vi "UnscentedKalmanFilter_Correct_OnlyUYR.vi"(4 "H_ExtraData":variant, 6 "H":T1, 7 "Rows":i32, 8 "R":T2, 9 "Y":T2, 10 "U":T2, 11 "in UnscentedKalmanFiilter":T3) -> (0 "Error":bool, 3 "out UnscentedKalmanFiilter":T3)   [LabVIEW 2019, in "Trajectory_Library.lvlib"]
doc: "Creates a new LINEAR SYSTEM data cluster with the specified values. \n\n\nInputs: \n - XXX -- XXX.\n\nOutputs:\n - XXX -- XXX."
uses:
  Trajectory_Library.lvlib
  UNSCENTED_KALMAN_FILTER.ctl
  <vilib>/Analysis/Matrix/Datatypes/RealMatrix.ctl
  MERWE_SCALED_SIGMA_PTS.ctl
  BiFunction_FUNC_TYPE.ctl
  <vilib>/Analysis/Matrix/NI_Matrix.lvlib
panel:
  # "<Inputs, 1>"
  # "<Rows, 1>"
  # "<Rows, Rows>"
  # "State Estimate <Statess,1>"
  # "<States, States>"
  # "<States, ?>"
  # "<Statess,  States>"
  # "<Outputs, Outputs>"
  # "<?, 1>"
  # "<?, 1>"
  # "State Estimate <Statess,1>"
  # "<States, States>"
  # "<States, ?>"
  # "<Statess,  States>"
  # "<Outputs, Outputs>"
  # "<?, 1>"
  # "<?, 1>"
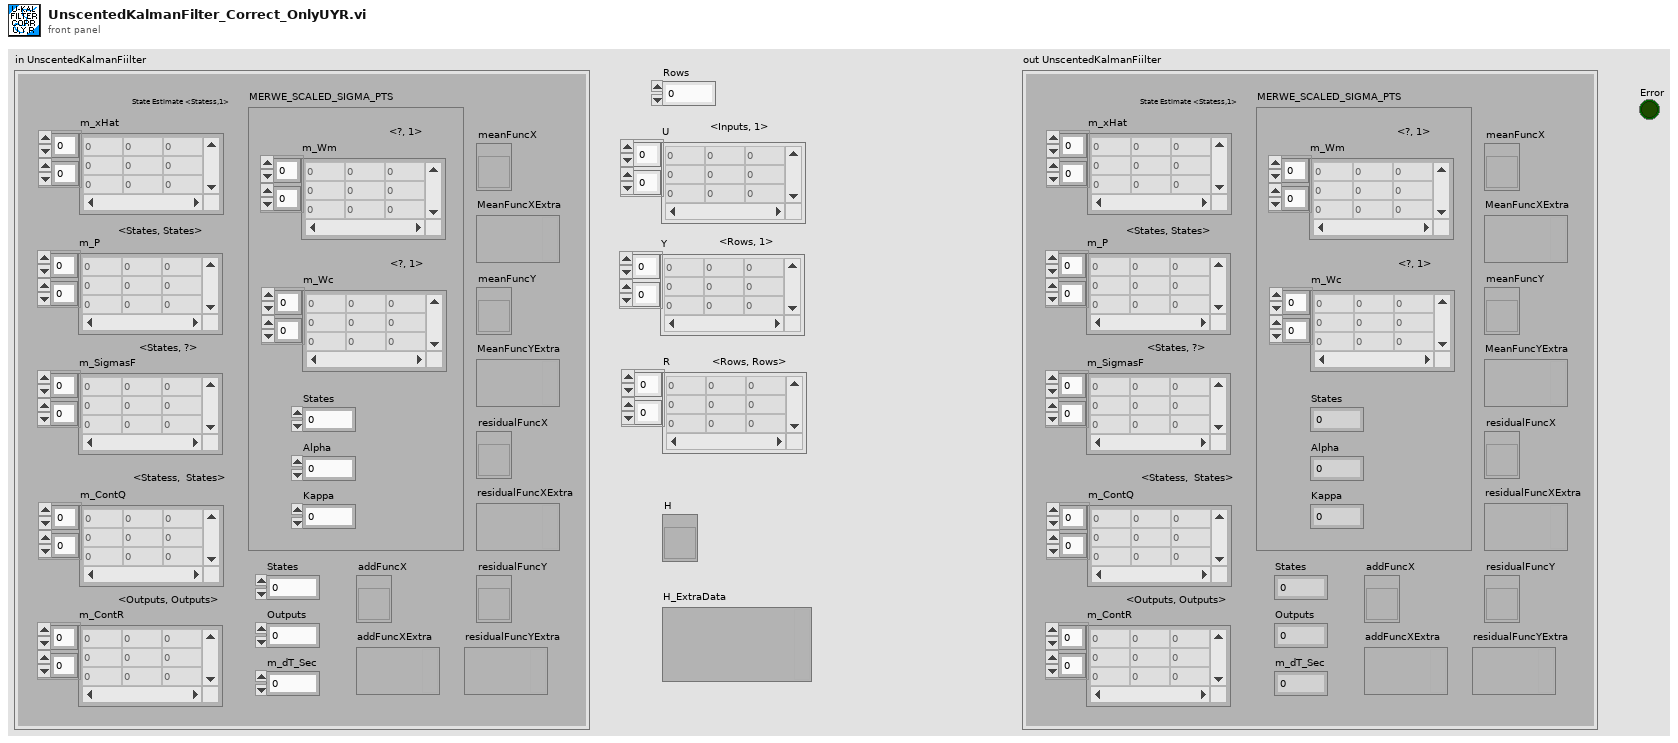
[diagram p1: front panel]
types:
  T1 = typedef "Trajectory_Library.lvlib/BiFunction_FUNC_TYPE.ctl" = refnum<vi>
  T2 = typedef "NI_Matrix.lvlib/RealMatrix.ctl" = dbl[][]
  T3 = typedef "Trajectory_Library.lvlib/UNSCENTED_KALMAN_FILTER.ctl" = cluster{"m_P":T2, "m_xHat":T2, "States":i32, "Outputs":i32, "m_ContR":T2, "m_ContQ":T2, "m_SigmasF":T2, "m_dT_Sec":dbl, "MERWE_SCALED_SIGMA_PTS":T4, "meanFuncX":T1, "meanFuncY":T1, "residualFuncX":T1, "residualFuncY":T1, "addFuncX":T1, "addFuncXExtra":variant, "residualFuncYExtra":variant, "residualFuncXExtra":variant, "MeanFuncYExtra":variant, "MeanFuncXExtra":variant}
  T4 = typedef "Trajectory_Library.lvlib/MERWE_SCALED_SIGMA_PTS.ctl" = cluster{"m_Wm":T2, "States":i32, "Alpha":dbl, "m_Wc":T2, "Kappa":i32}
  T5 = typedef "Trajectory_Library.lvlib/UNSCENTED_KALMAN_CORRECT_FUNC_GROUP.ctl" = cluster{"H_Func":T1, "meanFuncY":T1, "residualFuncY":T1, "residualFuncX":T1, "addFuncX":T1, "H_FuncExtra":variant, "MeanFuncYExtra":variant, "residualFuncYExtra":variant, "residualFuncXExtra":variant, "addFuncXExtra":variant}
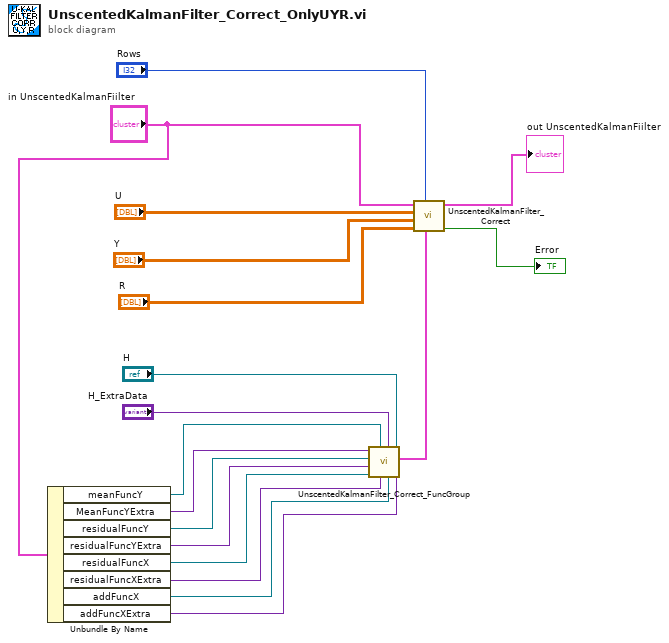
[diagram p0: block diagram]
diagram:
  n1 = Unbundle By Name("in UnscentedKalmanFiilter") -> ("meanFuncY"=w8:T1, "MeanFuncYExtra"=w7:variant, "residualFuncY"=w6:T1, "residualFuncYExtra"=w5:variant, "residualFuncX"=w4:T1, "residualFuncXExtra"=w3:variant, "addFuncX"=w2:T1, "addFuncXExtra"=w1:variant)
  n2 = call "UnscentedKalmanFilter_Correct_FuncGroup.vi"("addFuncXExtra"=w1, "H_Func"="H", "AddFuncX"=w2, "H_FuncExtra"="H_ExtraData", "residualFuncXExtra"=w3, "MeanFuncY"=w8, "ResidualFuncX"=w4, "residualFuncYExtra"=w5, "ResidualFuncY"=w6, "MeanFuncYExtra"=w7) -> ("UNSCENTED_KALMAN_CORRECT_FUNC_GROUP"=w12:T5)  [unwired: 1 in]
  n3 = call "UnscentedKalmanFilter_Correct.vi"("UNSCENTED_KALMAN_CORRECT_FUNC_GROUP"=w12, "Rows"="Rows", "R"="R", "Y"="Y", "U"="U", "in UnscentedKalmanFiilter"="in UnscentedKalmanFiilter") -> ("Error"=→"Error":bool, "out UnscentedKalmanFiilter"=→"out UnscentedKalmanFiilter":T3)  [unwired: 4 in]
